vi "IMAQ Type to MSC Type.vi"(0 "IMAQ Type":T1 items=["Grayscale (U8)", "Grayscale (I16)", "Grayscale (SGL)", "Complex (CSG)", "RGB (U32)", "HSL (U32)", "RGB (U64)", "Grayscale (U16)"], 11 "error in (no error)":errorcluster) -> (4 "Image TypeMSC Picture Type":T2 items=["Grayscale U8"=0, "Grayscale U16"=2, "Grayscale Single"=5, "Grayscale Double"=6, "RGB U8"=16], 15 "error out":errorcluster)   [LabVIEW 2014]
doc: "Conversion from IMAQ type to MSC Picture type"
uses:
  MSC Image_class/controls/Image Type.ctl
  MSC Image_class/MSC Image.lvclass
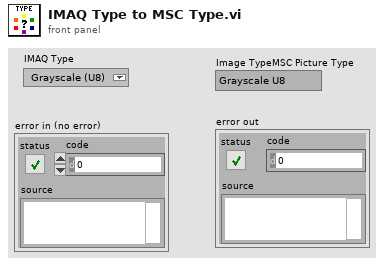
[diagram p1: front panel]
types:
  T1 = typedef "Image Type" = u32
  T2 = typedef "MSC Image.lvclass/Image Type.ctl" = i32
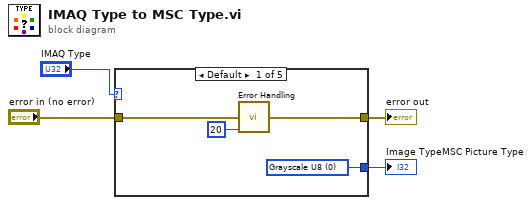
[diagram p0: block diagram]
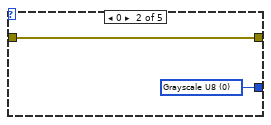
[diagram p2: hidden frame]
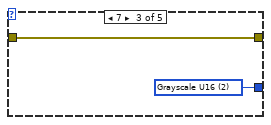
[diagram p3: hidden frame]
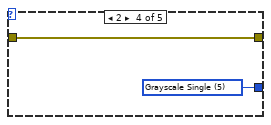
[diagram p4: hidden frame]
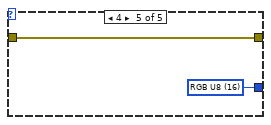
[diagram p5: hidden frame]
diagram:
  n1 = case shown="Default" "IMAQ Type" {
    tunnel: "error in (no error)" -> [w6 w10 w12 w14 w16]
    tunnel: [w8 w9 w11 w13 w15] -> w1
    tunnel: [w5 w10 w12 w14 w16] -> w3
    frame Default {
      w8 = T2 0 items=["Grayscale U8"=0, "Grayscale U16"=2, "Grayscale Single"=5, "Grayscale Double"=6, "RGB U8"=16] ("MSC Picture Type")
      n2 = call "Error Handling.vi"("error in (no error)"=w6, "return type"=20 ("code")) -> ("error out"=w5:errorcluster)  [unwired: 12 in, 1 out]
    }
    frame 0 {
      w9 = T2 0 items=["Grayscale U8"=0, "Grayscale U16"=2, "Grayscale Single"=5, "Grayscale Double"=6, "RGB U8"=16] ("MSC Picture Type")
    }
    frame 7 {
      w11 = T2 2 items=["Grayscale U8"=0, "Grayscale U16"=2, "Grayscale Single"=5, "Grayscale Double"=6, "RGB U8"=16] ("MSC Picture Type")
    }
    frame 2 {
      w13 = T2 5 items=["Grayscale U8"=0, "Grayscale U16"=2, "Grayscale Single"=5, "Grayscale Double"=6, "RGB U8"=16] ("MSC Picture Type")
    }
    frame 4 {
      w15 = T2 16 items=["Grayscale U8"=0, "Grayscale U16"=2, "Grayscale Single"=5, "Grayscale Double"=6, "RGB U8"=16] ("MSC Picture Type")
    }
  }
  "Image TypeMSC Picture Type" <- w1
  "error out" <- w3
